vi "报警信息记录.vi"(6 "platform_alarm_code":string, 7 "参数":string="质控单元", 8 "error in (no error)":errorcluster, 9 "code":u64, 10 "报警信息":string, 11 "Slave ID":T2=enum."氨氮") -> (0 "error out":errorcluster)   [LabVIEW 2016, in "质控单元V4.lvlib"]
panel:
  in  "data":T1={"时间"=timestamp(0 s since 1904-01-01), "参数"="水样测试", "元器件"="N", "故障现象"="", "故障分析"="", "state"="", "code"="", "platform_alarm_code"=""}
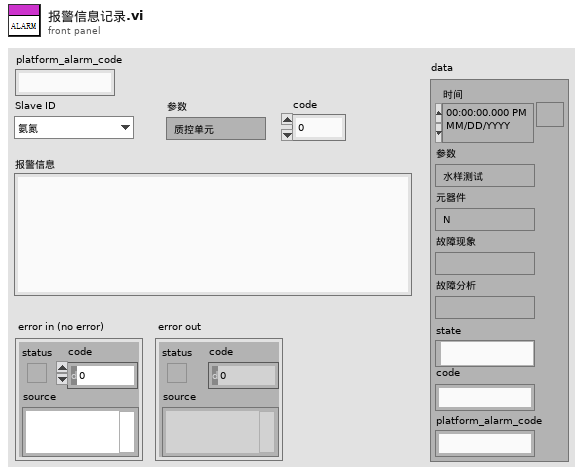
[diagram p1: front panel]
types:
  T1 = typedef "报警信息字段定义.ctl" = cluster{"时间":timestamp, "参数":string, "元器件":string, "故障现象":string, "故障分析":string, "state":string, "code":string, "platform_alarm_code":string}
  T2 = typedef "质控单元V4.lvlib/质控slave id.ctl" = enum16{"null", "氨氮", "总磷", "总氮", "CODMn", "CODCr", "氟化物"}
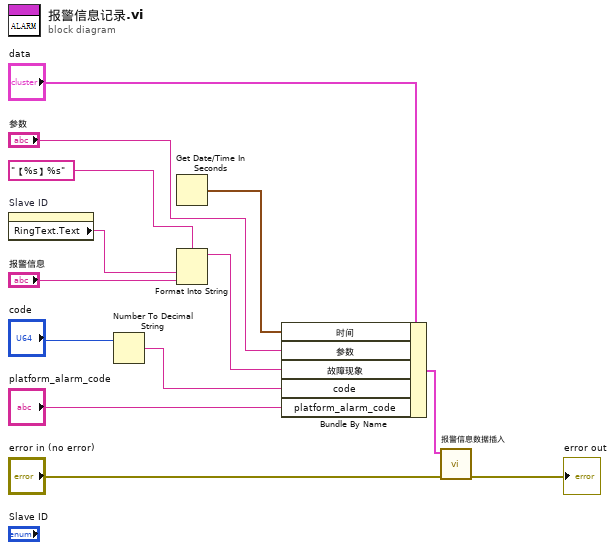
[diagram p0: block diagram]
diagram:
  n1 = property on="Slave ID" class="Enum (严格)"() -> ("RingText.Text"=w3:string)  [unwired: 2 in, 2 out]
  n2 = Number To Decimal String(number="code") -> (decimal integer string=w1:string)  [unwired: 1 in]
  n3 = Get Date/Time In Seconds() -> (seconds since 1Jan1904=w13:timestamp)
  n4 = Format Into String(format string="【%s】%s" ("格式字符串"), w3, "报警信息") -> (resulting string=w7:string)  [unwired: 2 in, 1 out]
  n5 = Bundle By Name(cluster="data", "时间"=w13, "参数"="参数", "故障现象"=w7, "code"=w1, "platform_alarm_code"="platform_alarm_code") -> (w11:T1)
  n6 = call "报警信息数据插入.vi"("data"=w11, "错误输入（无错误）"="error in (no error)") -> ("错误输出"=→"error out":errorcluster)  [unwired: 8 in]
